vi "_Unregister.vi"(8 "Error In":errorcluster, 10 "Listener ID":string, 11 "Listeners In":refnum<queue>[](array[refnum])) -> (0 "Error Out":errorcluster, 3 "Listeners Out":refnum<queue>[](array[refnum]))   [LabVIEW 2014, in "Logger.lvlib"]
uses:
  Logger.lvlib
  Public/Controls/Message.ctl
  Public/Controls/Tag.ctl
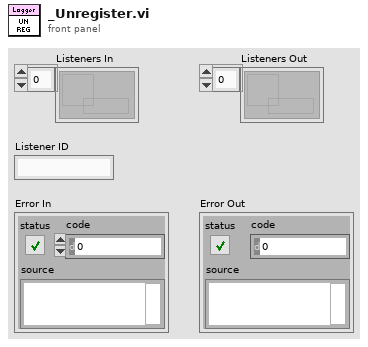
[diagram p1: front panel]
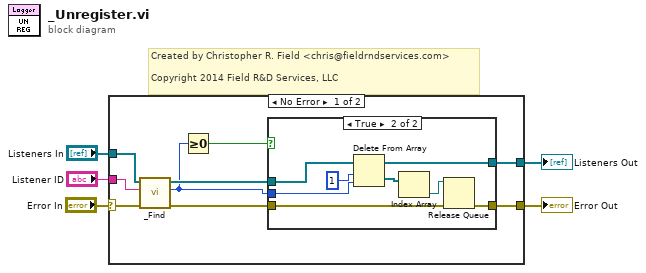
[diagram p0: block diagram]
diagram:
  # "Created by Christopher R. Field <chris@fieldrndservices.com>\n\nCopyright 2014 Field R&D Services, LLC"
  n1 = case shown="No Error" "Error In" {
    selector: "Error In" -> [w7 w25]
    tunnel: [w14 w25] -> w5
    tunnel: [w13 w26] -> w4
    tunnel: "Listeners In" -> [w11 w26]
    tunnel: "Listener ID" -> [w8 _]
    frame No Error {
      n2 = call "_Find.vi"("Error In"=w7, "Listener ID"=w8, "Listeners In"=w11) -> ("Error Out"=w6:errorcluster, "Index"=w9:i32, "Listeners Out"=w10:refnum<queue>[])  [unwired: 6 in]
      n3 = Greater Or Equal To 0?(x=w9) -> (x >= 0?=w12:bool)
      n4 = case shown="True" w12 {
        tunnel: w10 -> [w16 w24]
        tunnel: w9 -> [_ w22]
        tunnel: [w16 w21] -> w13
        tunnel: w6 -> [w15 w18]
        tunnel: [w15 w17] -> w14
        frame False {
        }
        frame True {
          n5 = Delete From Array(array=w24, length=1, index=w22) -> (deleted portion=w20:refnum<queue>[], array with subset deleted=w21:refnum<queue>[])
          n6 = Index Array(array=w20) -> (element=w19:refnum<queue>)  [unwired: 1 in]
          n7 = Release Queue(queue=w19, error in (no error)=w18) -> (error out=w17:errorcluster)  [unwired: 1 in, 2 out]
        }
      }
    }
    frame Error {
    }
  }
  "Error Out" <- w5
  "Listeners Out" <- w4
